vi "Fields Strip Spartan SN Prefix.vi"(1 "Spartan SN":string) -> (0 "Stripped Spartan SN":string)   [LabVIEW 2011]
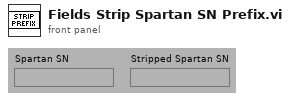
[diagram p1: front panel]
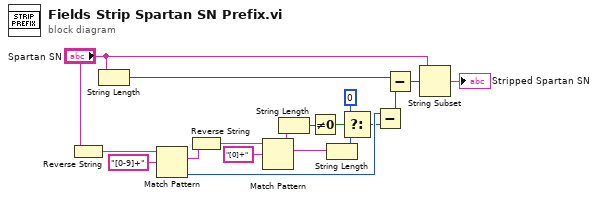
[diagram p0: block diagram]
diagram:
  n1 = Reverse String(1:"Spartan SN") -> (0:w18:string)
  n2 = String Length(string="Spartan SN") -> (length=w16:i32)
  n3 = Match Pattern(string=w18, regular expression="[0-9]+") -> (match substring=w10:string, offset past match=w12:i32)  [unwired: 3 out]
  n4 = Reverse String(1:w10) -> (0:w14:string)
  n5 = Match Pattern(string=w14, regular expression="[0]+") -> (before substring=w9:string, match substring=w13:string)  [unwired: 3 out]
  n6 = String Length(string=w9) -> (length=w8:i32)
  n7 = Not Equal To 0?(x=w8) -> (x != 0?=w7:bool)
  n8 = String Length(string=w13) -> (length=w6:i32)
  n9 = Select(t=0, s=w7, f=w6) -> (s? t:f=w3:i32)
  n10 = Subtract(x=w12, y=w3) -> (x-y=w11:i32)
  n11 = Subtract(x=w16, y=w11) -> (x-y=w4:i32)
  n12 = String Subset(string="Spartan SN", offset (0)=w4) -> (substring=→"Stripped Spartan SN":string)  [unwired: 1 out]
